vi "Read connection ID.vi"(8 "error in (no error)":errorcluster, 11 "Connection.TCP":refnum<class "Connection.TCP.lvclass">) -> (0 "error out":errorcluster, 1 "outbound":refnum<k5>, 2 "inbound":refnum<k5>, 3 "Connection.TCP":refnum<class "Connection.TCP.lvclass">)   [LabVIEW 2013, in "Connection.TCP_GOSPL.lvlib" / "Connection.TCP.lvclass"]
uses:
  Connection.TCP.lvclass
  Connection.TCP.lvclass/Connection.TCP.ctl
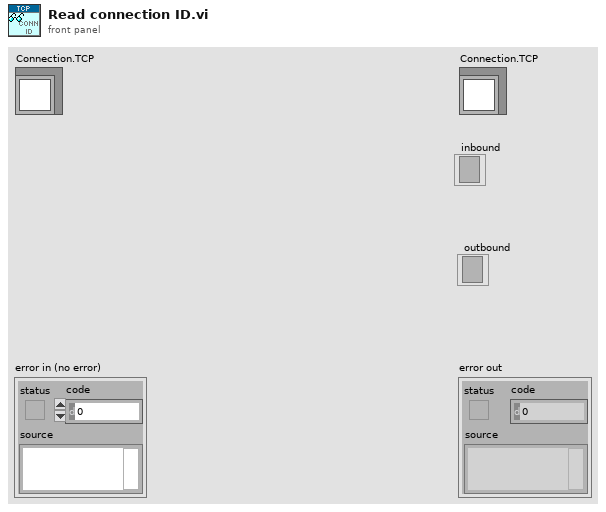
[diagram p1: front panel]
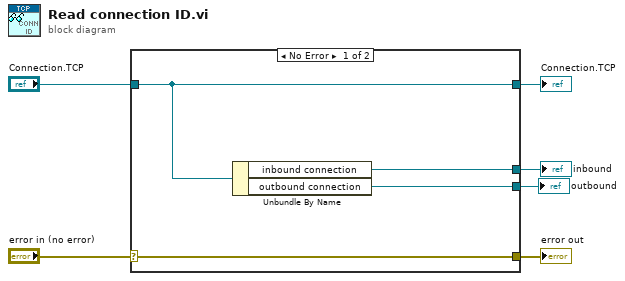
[diagram p0: block diagram]
diagram:
  n1 = case shown="No Error" "error in (no error)" {
    selector: "error in (no error)" -> [w10 w11]
    tunnel: [w10 w11] -> w5
    tunnel: [w9 w12] -> w3
    tunnel: "Connection.TCP" -> [w9 w12]
    tunnel: [w8 _] -> w2
    tunnel: [w7 _] -> w1
    frame No Error {
      n2 = Unbundle By Name(w9) -> ("inbound connection"=w8:refnum<k5>, "outbound connection"=w7:refnum<k5>)
    }
    frame Error {
    }
  }
  "error out" <- w5
  "Connection.TCP" <- w3
  "inbound" <- w2
  "outbound" <- w1
